vi "New.vi"(4 "Buffers":refnum<class "Buffers.lvclass">, 5 "FIFO Options":T2, 6 "thread settings":T1={"Priority"=100, "Processor"=-2, "ID"=0}, 7 "Plugin Interfaces Pool":refnum<class "Plugin Interface Pool.lvclass">, 8 "error in (no error)":errorcluster, 9 "Transfer Groups":refnum<class "Transfer Group.lvclass">[](array[class]), 10 "Buffer Converter":refnum<class "Buffer Converter.lvclass">, 11 "Transceiver":refnum<class "Transceiver.lvclass">) -> (0 "error out":errorcluster, 2 "Plugin Thread Interface":refnum<class "Plugin Interface.lvclass">, 3 "Plugin Thread out":refnum<class "Plugin Thread.lvclass">)   [LabVIEW 2017, in "DSF Core.lvlib" / "Plugin Thread.lvclass"]
uses:
  Thread/Plugin/Plugin Thread.lvclass
  C:/Users/Admin/Desktop/Data Sharing Framework/Source/Core/Classes/Thread/Thread.lvclass
  Transceiver.lvclass
  Typedefs/DSF FIFO Options.ctl
  Transfer Group/Transfer Group.lvclass
  Buffer Converter/Buffer Converter.lvclass
  Thread Pool/Plugin Interface Pool.lvclass
  C:/Users/Admin/Desktop/Data Sharing Framework/Source/Core/Classes/Thread Pool/Pool.lvclass
  Thread/Thread Settings.ctl
  Interfaces/Transceiver Interface/Plugin Interface.lvclass
  C:/Users/Admin/Desktop/Data Sharing Framework/Source/Core/Classes/Interfaces/Interface/Interface.lvclass
  Buffer/Buffers.lvclass
  Thread Pool/Plugin Interface Pool.lvclass/Plugin Interface Pool.ctl
  Thread Pool/Pool.lvclass/Pool.ctl
  Interfaces/Interface/Interface.lvclass/Interface.ctl
  Thread/Thread.lvclass/Thread.ctl
  Thread/Plugin/Plugin Thread.lvclass/Plugin Thread.ctl
  Thread Pool/Read FIFO.vi
  Thread Pool/Write FIFO.vi
  Thread/Thread.lvclass
  Interfaces/Interface/Interface.lvclass
  DSF Core.lvlib
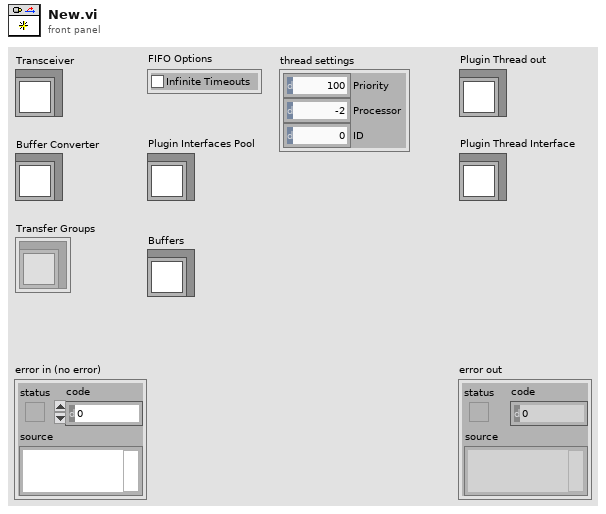
[diagram p1: front panel]
types:
  T1 = typedef "DSF Core.lvlib/Thread.lvclass/Thread Settings.ctl" = cluster{"Priority":u16, "Processor":i32, "ID":i32}
  T2 = typedef "DSF Core.lvlib/DSF FIFO Options.ctl" = cluster{"Infinite Timeouts":bool}
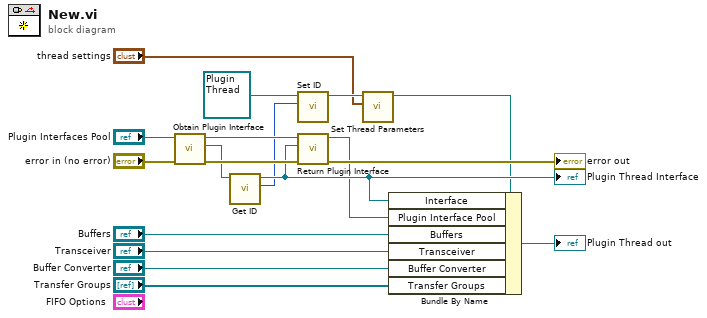
[diagram p0: block diagram]
diagram:
  n1 = call "Obtain Plugin Interface.vi"("error in (no error)"="error in (no error)", "Plugin Interface Pool in"="Plugin Interfaces Pool") -> ("error out"=w18:errorcluster, "Plugin Interface"=w6:refnum<class "Plugin Interface.lvclass">, "Plugin Interface Pool out"=w5:refnum<class "Plugin Interface Pool.lvclass">)  [unwired: 6 in, 1 out]
  n2 = call "Get ID.vi"("Interface in"=w6) -> ("ID"=w1:i32, "Interface out"=w4:refnum<class "Plugin Interface.lvclass">)  [unwired: 9 in]
  "Plugin Thread Interface" <- w4
  n3 = call "Set ID.vi"("id"=w1, "Thread in"=refnum<class "Plugin Thread.lvclass"> refnum ("Transceiver Thread in")) -> ("Thread out"=w14:refnum<class "Plugin Thread.lvclass">)  [unwired: 9 in]
  n4 = call "Return Plugin Interface.vi"("error in (no error)"=w18, "Plugin Interface"=w4, "Plugin Interface Pool in"=w5) -> ("error out"=→"error out":errorcluster, "Plugin Interface Pool out"=w3:refnum<class "Plugin Interface Pool.lvclass">)  [unwired: 6 in, 1 out]
  n5 = call "Set Thread Parameters.vi"("thread settings"="thread settings", "Thread in"=w14) -> ("Thread out"=w2:refnum<class "Plugin Thread.lvclass">)  [unwired: 9 in]
  n6 = Bundle By Name(cluster=w2, "Interface"=w4, "Plugin Interface Pool"=w3, "Buffers"="Buffers", "Transceiver"="Transceiver", "Buffer Converter"="Buffer Converter", "Transfer Groups"="Transfer Groups") -> (→"Plugin Thread out":refnum<class "Plugin Thread.lvclass">)
